vi "Write message.vi"(8 "error in (no error)":errorcluster, 9 "Write request":T1, 10 "timeout ms (1000)":i32, 11 "WAMP Client in":refnum<class "WAMP Client.lvclass">) -> (0 "error out":errorcluster, 3 "WAMP Client out":refnum<class "WAMP Client.lvclass">)   [LabVIEW 2020, in "wamplv.lvlib" / "WAMP Client.lvclass"]
uses:
  WAMP Client.lvclass
  WAMP Client.lvclass/WAMP Client.ctl
  Private/Comm Handlers/ICommHandler/ICommHandler.lvclass
  Private/TypeDefs/Transport type.ctl
  wamplv.lvlib
  TypeDef/Write queue item.ctl
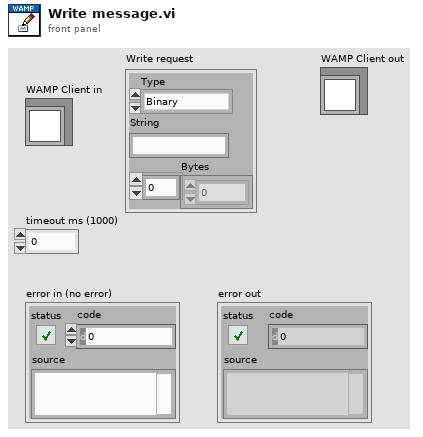
[diagram p1: front panel]
types:
  T1 = typedef "wamplv.lvlib/Write queue item.ctl" = cluster{"Type":T2, "String":string, "Bytes":u8[]}
  T2 = typedef "wamplv.lvlib/Transport type.ctl" = enum16{"Binary", "Text"}
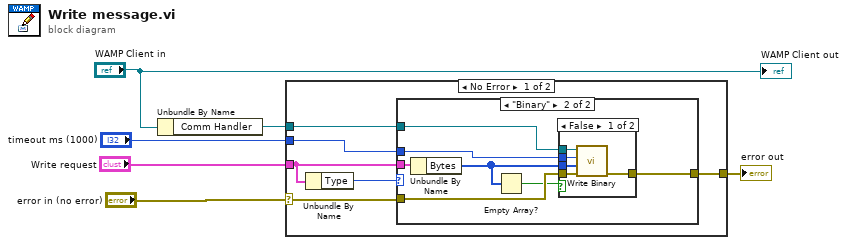
[diagram p0: block diagram]
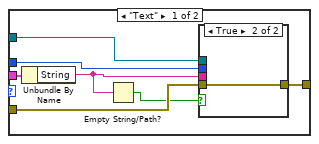
[diagram p2: hidden frame]
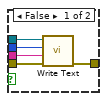
[diagram p3: hidden frame]
diagram:
  n1 = Unbundle By Name("WAMP Client in") -> ("Comm Handler"=w5:refnum<class "ICommHandler.lvclass">)
  n2 = case shown="No Error" "error in (no error)" {
    selector: "error in (no error)" -> [w11 w39]
    tunnel: "timeout ms (1000)" -> [w9 _]
    tunnel: w5 -> [w10 _]
    tunnel: [w12 w39] -> w3
    tunnel: "Write request" -> [w7 _]
    frame No Error {
      n3 = Unbundle By Name(w7) -> ("Type"=w8:T2)
      n4 = case shown="\"Binary\"" w8 {
        tunnel: [w19 w31] -> w12
        tunnel: w11 -> [w18 w30]
        tunnel: w10 -> [w17 w28]
        tunnel: w9 -> [w16 w29]
        tunnel: w7 -> [w15 w32]
        frame "Text" {
          n5 = Unbundle By Name(w15) -> ("String"=w14:string)
          n6 = Empty String/Path?(string/path=w14) -> (empty?=w13:bool)
          n7 = case shown="True" w13 {
            tunnel: [w24 w25] -> w19
            tunnel: w18 -> [w23 w25]
            tunnel: w17 -> [w22 _]
            tunnel: w16 -> [w21 _]
            tunnel: w14 -> [w20 _]
            frame False {
              n8 = call-dynamic "Write Text.vi"("error in (no error)"=w23, "String"=w20, "timeout ms (1000)"=w21, "ICommHandler in"=w22) -> ("error out"=w24:errorcluster)  [unwired: 6 in, 1 out]
            }
            frame True {
            }
          }
        }
        frame "Binary" {
          n9 = Unbundle By Name(w32) -> ("Bytes"=w27:u8[])
          n10 = Empty Array?(array=w27) -> (empty?=w26:bool)
          n11 = case shown="False" w26 {
            tunnel: [w37 w38] -> w31
            tunnel: w30 -> [w36 w38]
            tunnel: w29 -> [w35 _]
            tunnel: w28 -> [w34 _]
            tunnel: w27 -> [w33 _]
            frame False {
              n12 = call-dynamic "Write Binary.vi"("error in (no error)"=w36, "Bytes"=w33, "timeout ms (1000)"=w35, "ICommHandler in"=w34) -> ("error out"=w37:errorcluster)  [unwired: 4 in, 1 out]
            }
            frame True {
            }
          }
        }
      }
    }
    frame Error {
    }
  }
  "error out" <- w3
  "WAMP Client out" <- "WAMP Client in"
